vi "Slide Callback.vi"(7 "Owner":refnum<class>, 11 "Message":refnum<class "Message.lvclass">) -> (0 "error out":errorcluster)   [LabVIEW 2020]
uses:
  Stream-Simple-Msg/Message/Message.lvclass
  56a5a06d-eb56-4e44-b9be-13e5cc0f8f90.vi
  Stream-Simple-Msg/Message/Get Data.vi
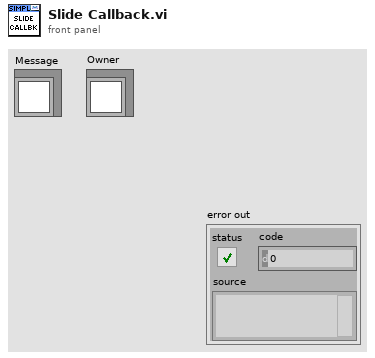
[diagram p1: front panel]
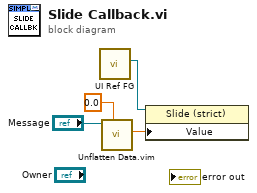
[diagram p0: block diagram]
diagram:
  n1 = call "UI Ref FG.vi"() -> ("Slide"=w3:refnum<vi>)  [unwired: 9 in, 2 out]
  n2 = call "Unflatten Data.vim"("Data Type"=0.0, "Message in"="Message") -> ("Unflattened Data"=w2:dbl)  [unwired: 7 in, 2 out]
  n3 = property class="Slide (strict)"(reference=w3, "Value"=w2) -> ()  [unwired: 1 in, 2 out]
